vi "Create.vi"(8 "error in (no error)":errorcluster, 10 "source pointer":i64, 11 "Source in":refnum<class "Source.lvclass">) -> (0 "error out":errorcluster, 3 "Source out":refnum<class "Source.lvclass">)   [LabVIEW 2020, in "Server.lvlib" / "Source.lvclass"]
uses:
  Source.lvclass
  Source.lvclass/Source.ctl
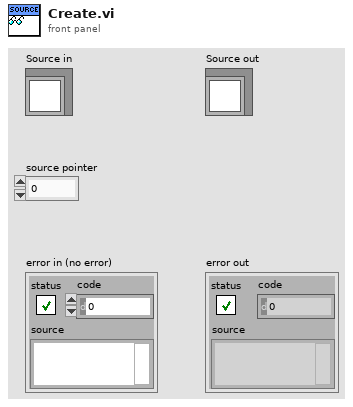
[diagram p1: front panel]
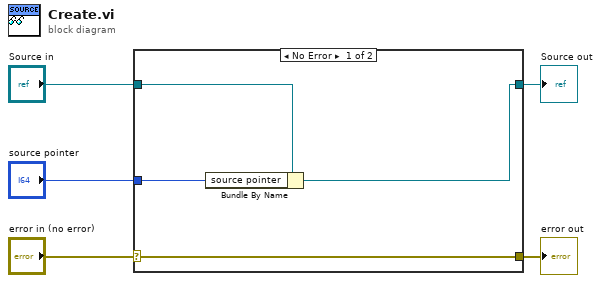
[diagram p0: block diagram]
diagram:
  n1 = case shown="No Error" "error in (no error)" {
    selector: "error in (no error)" -> [w9 w10]
    tunnel: [w9 w10] -> w4
    tunnel: [w7 w11] -> w2
    tunnel: "Source in" -> [w8 w11]
    tunnel: "source pointer" -> [w6 _]
    frame No Error {
      n2 = Bundle By Name(cluster=w8, "source pointer"=w6) -> (w7:refnum<class "Source.lvclass">)
    }
    frame Error {
    }
  }
  "error out" <- w4
  "Source out" <- w2
